vi "4310 Reset Device.vi"() -> ()   [LabVIEW 2019]
panel:
  out "Numeric Control":dbl
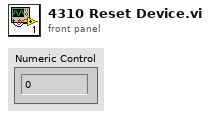
[diagram p1: front panel]
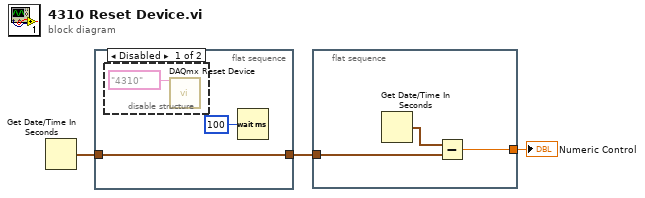
[diagram p0: block diagram]
diagram:
  n1 = Get Date/Time In Seconds() -> (seconds since 1Jan1904=w3:timestamp)
  n2 = flat-sequence {
    tunnel: w3 -> [w5]
    tunnel: [w5] -> w2
    frame #0 {
      n3 = disable-structure shown="Disabled" {
        frame Disabled {
          n4 = call <vilib>:"DAQmx Reset Device.vi"("device in"=tag "4310") -> ()  [unwired: 14 in, 1 out]
        }
        frame Enabled {
        }
      }
      n5 = Wait (ms)(milliseconds to wait=u32 100) -> ()  [unwired: 1 out]
    }
  }
  n6 = flat-sequence {
    tunnel: w2 -> [w8]
    tunnel: [w7] -> w1
    frame #0 {
      n7 = Get Date/Time In Seconds() -> (seconds since 1Jan1904=w9:timestamp)
      n8 = Subtract(x=w9, y=w8) -> (x-y=w7:dbl)
    }
  }
  "Numeric Control" <- w1
